vi "FTP List Directories.vi"(6 "Base Path":string, 7 "Remote Port":u16=21, 8 "error in (no error)":errorcluster, 9 "Password":string, 10 "User":string, 11 "Server / IP Address":string) -> (0 "error out":errorcluster, 3 "dir list":T1[](array[typedef]))   [LabVIEW 2013]
doc: "Returns a list of the directories on the remote system under the specified base path.\n\n\nVersion 1.0 - 02/13/2013\n\nPhaeron, Inc.\nwww.phaeron.com\ninfo@phaeron.com"
uses:
  <vilib>/FTP/ftp2.llb/FTP File Info.ctl
  <vilib>/FTP/NI_FTP.lvlib
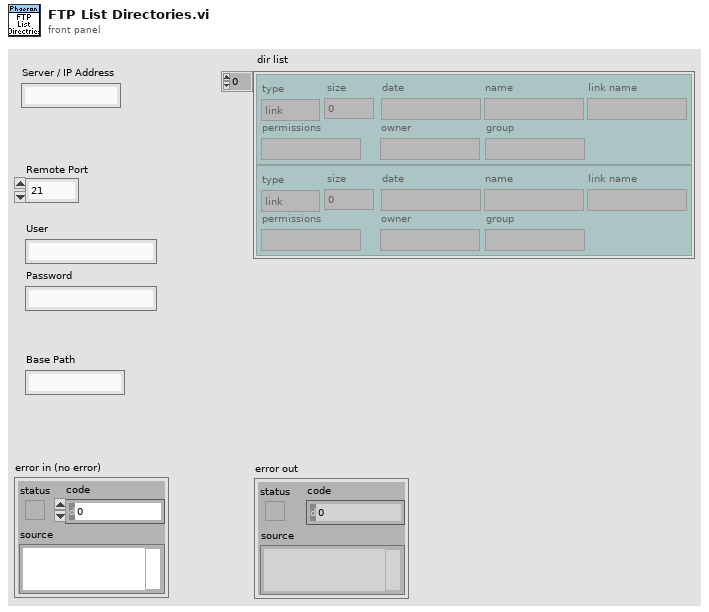
[diagram p1: front panel]
types:
  T1 = typedef "NI_FTP.lvlib/FTP File Info.ctl" = cluster{"type":enum16{"unknown", "file", "dir", "link"}, "permissions":string, "owner":string, "group":string, "size":i32, "date":string, "name":string, "link name":string}
  T2 = typedef "NI_FTP.lvlib/FTP Session.ctl" = refnum<k5>
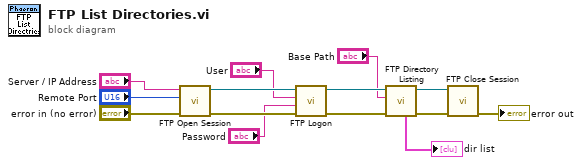
[diagram p0: block diagram]
diagram:
  n1 = call <vilib>:"FTP Open Session.vi"("error in (no error)"="error in (no error)", "remote port (21)"="Remote Port", "address"="Server / IP Address") -> ("error out"=w10:errorcluster, "ftp session"=w11:T2)  [unwired: 5 in, 2 out]
  n2 = call <vilib>:"FTP Logon.vi"("error in (no error)"=w10, "password"="Password", "user"="User", "ftp session"=w11) -> ("error out"=w12:errorcluster, "ftp session out"=w13:T2)  [unwired: 4 in, 2 out]
  n3 = call <vilib>:"FTP Directory Listing.vi"("error in (no error)"=w12, "directory path"="Base Path", "ftp session"=w13) -> ("error out"=w9:errorcluster, "ftp session out"=w7:T2, "dir list"=→"dir list":T1[])  [unwired: 4 in, 2 out]
  n4 = call <vilib>:"FTP Close Session.vi"("error in (no error)"=w9, "ftp session"=w7) -> ("error out"=→"error out":errorcluster)  [unwired: 6 in, 3 out]
